vi "Parse Nanovoltmeter Data.vi"(8 "error in":errorcluster, 11 "Data":string) -> (0 "error out":errorcluster, 2 "Voltages (V)":dbl[](array[numeric]) format="%#_9g", 3 "Relative times (s)":dbl[](array[numeric]) format="%#_9g", 4 "Std. Dev. (V)":dbl, 6 "Mean (V)":dbl)   [LabVIEW 2019, in "ACSVcontrol-driver.lvlib"]
doc: "Parse data recieved from PJVS with nanovoltmeter data."
uses:
  ACSVcontrol-driver.lvlib
  <vilib>/Utility/error.llb/Error Cluster From Error Code.vi
  <vilib>/regexp/Match Regular Expression.xnode
  <vilib>/ErrorRing/Error Ring.xnode
  <vilib>/Analysis/NI_AALBase.lvlib
panel:
  out "Waveform Graph":dbl[][](graph)
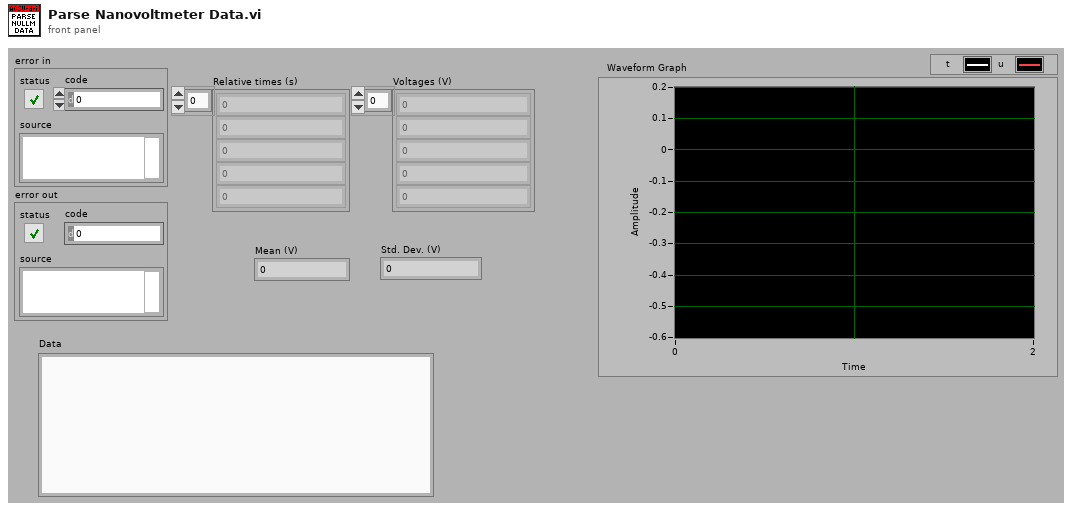
[diagram p1: front panel]
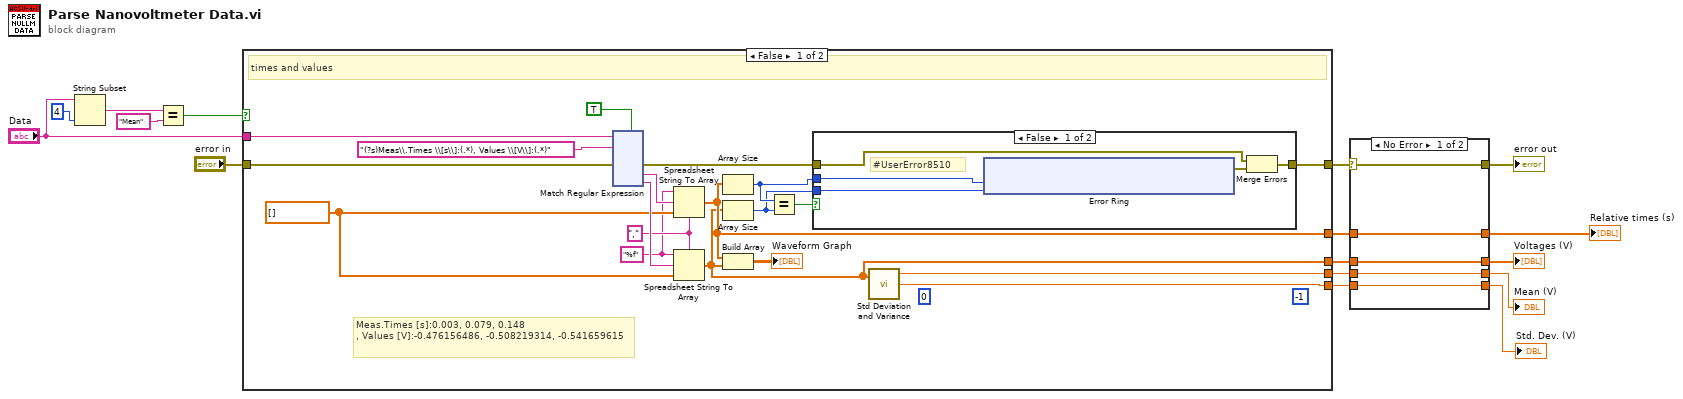
[diagram p0: block diagram]
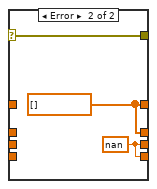
[diagram p2: hidden frame]
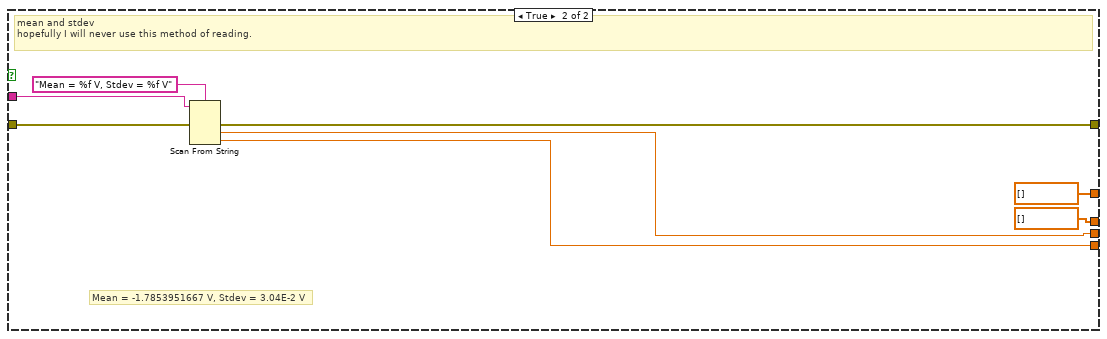
[diagram p4: hidden frame]
diagram:
  n1 = String Subset(string="Data", length (rest)=4 ("length (rest)")) -> (substring=w15:string)  [unwired: 1 in]
  n2 = Equal?(x=w15, y="Mean") -> (x = y?=w13:bool)
  n3 = case shown="False" w13 {
    tunnel: "Data" -> [w26 w173]
    tunnel: "error in" -> [w21 w172]
    tunnel: [w34 w171] -> w10
    tunnel: [w32 w170] -> w5
    tunnel: [w31 w169] -> w3
    tunnel: [w28 dbl[] [] ("array type (2D Dbl)")] -> w1
    tunnel: [w29 dbl[] [] ("array type (2D Dbl)")] -> w7
    frame False {
      w19 = dbl[] [] ("array type (2D Dbl)")
      (unwired) 0 ("line index")
      (unwired) -1 ("default value 1")
      w17 = "%f" ("format string")
      w18 = "," ("delimiter (Tab)")
      # "Meas.Times [s]:0.003, 0.079, 0.148\n, Values [V]:-0.476156486, -0.508219314, -0.541659615"
      # "times and values"
      n4 = xnode "Match Regular Expression"("input string"=w26, "regular expression"="(?s)Meas\\.Times \\[s\\]:(.*), Values \\[V\\]:(.*)", "error in"=w21, "multiline? (F)"=TRUE) -> ("error out"=w20:errorcluster, "submatch 1"=w22:string, "submatch 2"=w23:string)  [unwired: 2 in, 4 out]
      n5 = Spreadsheet String To Array(delimiter (Tab)=w18, format string=w17, spreadsheet string=w22, array type (2D Dbl)=w19) -> (array=w29:dbl[])
      n6 = Spreadsheet String To Array(delimiter (Tab)=w18, format string=w17, spreadsheet string=w23, array type (2D Dbl)=w19) -> (array=w28:dbl[])
      n7 = Array Size(array=w29) -> (size(s)=w33:i32)
      n8 = Array Size(array=w28) -> (size(s)=w30:i32)
      n9 = Build Array(w29, w28) -> (→"Waveform Graph":dbl[][])
      n10 = Equal?(x=w33, y=w30) -> (x = y?=w35:bool)
      n11 = case shown="False" w35 {
        tunnel: [w155 w166] -> w34
        tunnel: w20 -> [w156 w166]
        tunnel: w33 -> [w154 _]
        tunnel: w30 -> [w153 _]
        frame False {
          # "#UserError8510"
          n12 = xnode "Error Ring"("parameter 0"=w154, "parameter 1"=w153) -> ("error out"=w157:errorcluster)
          n13 = Merge Errors(w156, w157) -> (w155:errorcluster)
        }
        frame True {
        }
      }
      n14 = call <vilib>:"Std Deviation and Variance.vi"("X"=w28) -> ("mean"=w32:dbl, "standard deviation"=w31:dbl)  [unwired: 1 in, 1 out]
    }
    frame True {
      # "Mean = -1.7853951667 V, Stdev = 3.04E-2 V"
      # "mean and stdev\nhopefully I will never use this method of reading."
      n15 = Scan From String(format string="Mean = %f V, Stdev = %f V", input string=w173, error in=w172) -> (error out=w171:errorcluster, output 1=w170:dbl, output 2=w169:dbl)  [unwired: 3 in, 2 out]
    }
  }
  n16 = case shown="No Error" w10 {
    selector: w10 -> [w179 w182]
    tunnel: [w179 w182] -> w9
    tunnel: [w178 w181] -> w8
    tunnel: w7 -> [w178 _]
    tunnel: [w177 w180] -> w6
    tunnel: w5 -> [w177 _]
    tunnel: [w176 w180] -> w4
    tunnel: w3 -> [w176 _]
    tunnel: [w175 w181] -> w2
    tunnel: w1 -> [w175 _]
    frame No Error {
    }
    frame Error {
      w180 = nan
      w181 = dbl[] [] ("array type (2D Dbl)")
    }
  }
  "error out" <- w9
  "Mean (V)" <- w6
  "Std. Dev. (V)" <- w4
  "Voltages (V)" <- w2
  "Relative times (s)" <- w8
